vi "子VI-深度学习自动检测结果分析.vi"(2 "临界Z值":i32, 4 "临界面积百分比值":dbl, 6 "预测图片保存路径":path, 12 "产品规格":cluster{"产品长度（周长）（mm）":dbl, "产品宽度（母线长）（mm）":dbl}) -> (15 "全部检测结果":string[][](table), 16 "弥散类检测结果":string[][](table), 17 "Threshold Image":T2(plugin-control), 18 "misan":T2(plugin-control))   [LabVIEW 2018]
uses:
  <vilib>/vision/NI_Vision_Development_Module.lvlib
panel:
  out "?":string[][](table)
  in  "格式字符串 4":string="%f"
  in  "分隔符（'\\'代码显示） 3":string="\t"
  in  "Tab Control":T1
  out "?":T2(plugin-control)
  in  "格式字符串 3":string="%f"
  in  "分隔符（'\\'代码显示） 2":string="\t"
  out "弥散和分层临界灰度值":i64
  out "弥散缺陷个数":i32
  out "分层缺陷个数":i32
  out "合格？ 弥散类":string="fencengThreshold"
  out "合格？分层类":string="fencengThreshold"
  out "面积 (pixels)":i32
  in  "格式字符串 2":string="%f"
  in  "分隔符（'\\'代码显示）":string="\t"
  out "缺陷初步分类的临界值":sgl format="%#.3f"
  # "所选区域信息"
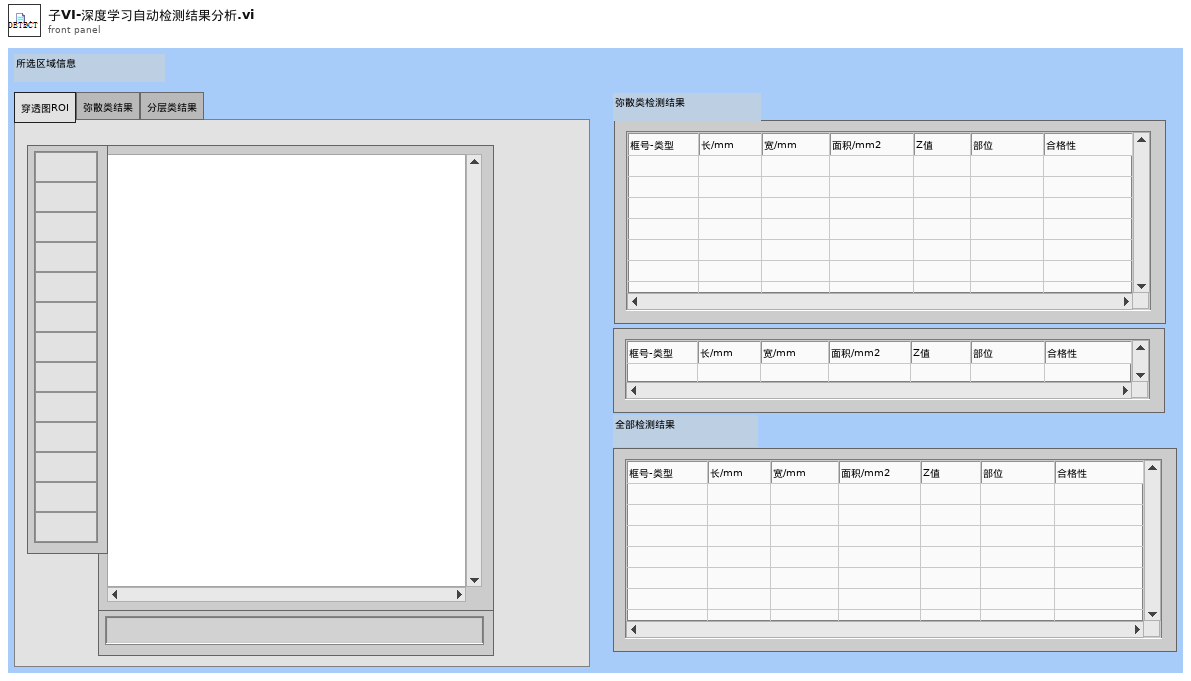
[diagram p1: front panel]
types:
  T1 = typedef "控件2.ctl" = enum32{"穿透图ROI", "弥散类结果", "分层类结果"}
  T2 = typedef "IMAQ Image.ctl" = refnum<image>
  T3 = typedef "Image Type" = u32
  T4 = typedef "Particle Parameters" = i32
  T5 = cluster{"Measurement Parameter":T4, "Range Lower Value":dbl, "Range Upper Value":dbl, "Range":bool, "Measurement Type":bool}[]
  T6 = cluster{"histogram":u32[], "Minimal Value":sgl, "Maximal Value":sgl, "Starting Value":sgl, "Interval Width":sgl, "Mean Value":sgl, "Standard  Variation":sgl, "Area (pixels)":i32}
  T7 = cluster{"Area":dbl, "Number of Holes":dbl, "Bounding Rect":cluster{"Left":dbl, "Top":dbl, "Right":dbl, "Bottom":dbl}, "Center of Mass":cluster{"X":dbl, "Y":dbl}, "Orientation":dbl, "Dimensions":cluster{"Width":dbl, "Height":dbl}}[]
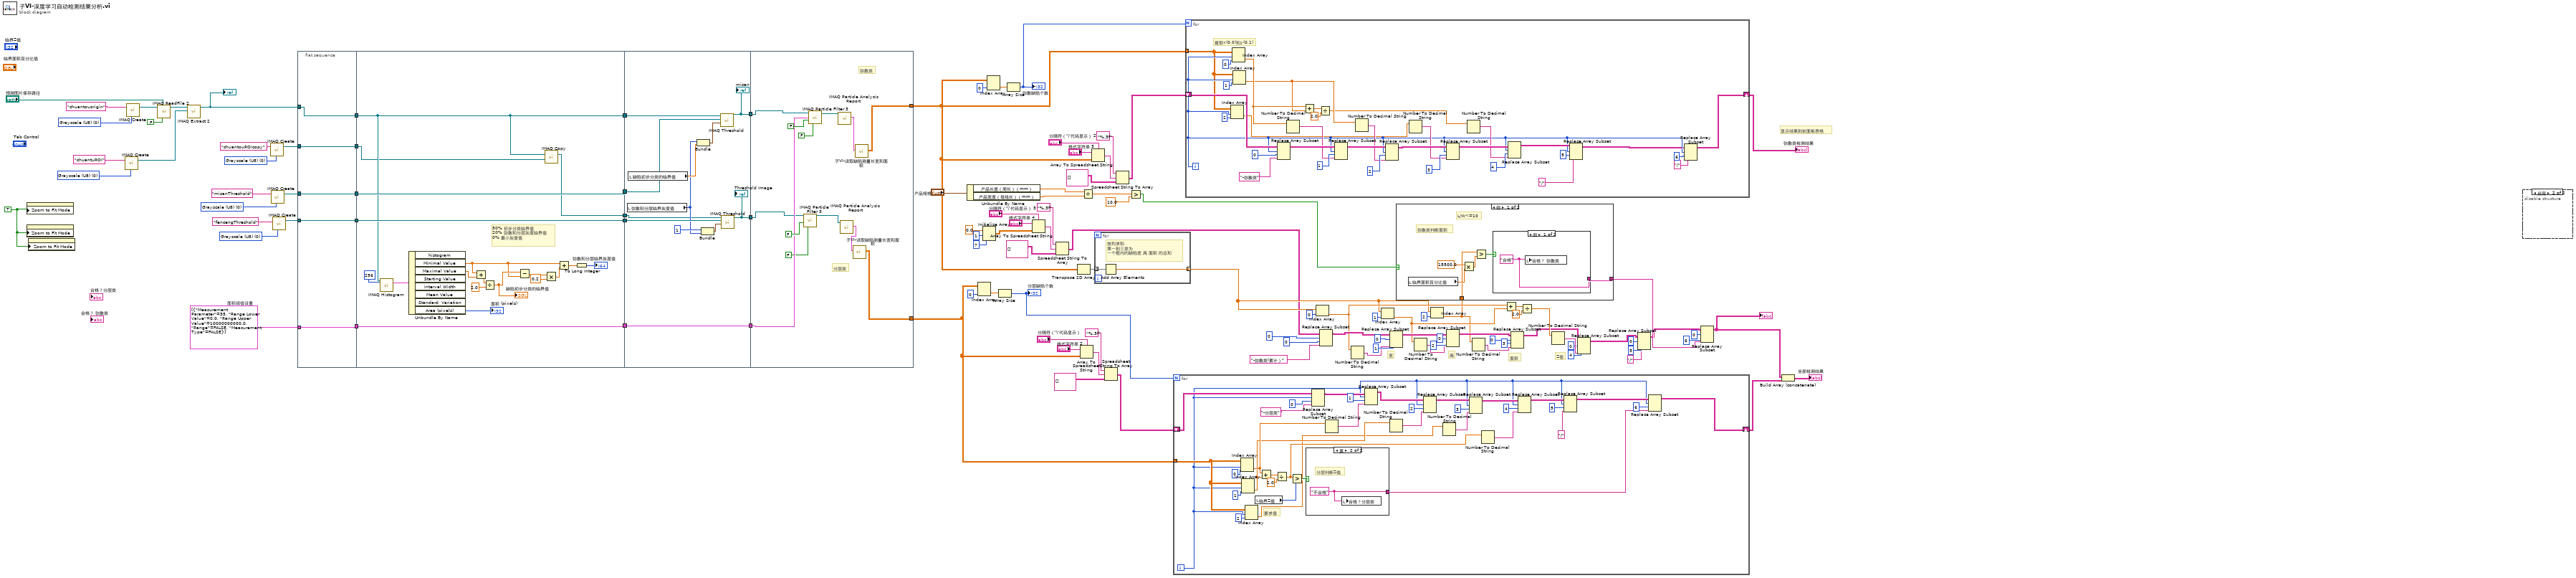
[diagram p0: block diagram]
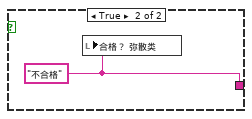
[diagram p2: hidden frame]
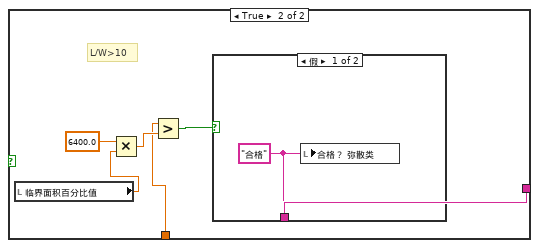
[diagram p3: hidden frame]
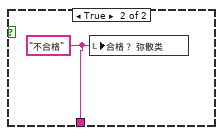
[diagram p4: hidden frame]
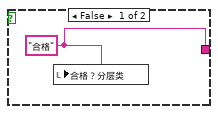
[diagram p5: hidden frame]
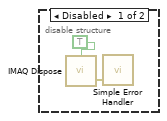
[diagram p6: hidden frame]
diagram:
  w55 = T3 0 items=["Grayscale (U8)", "Grayscale (I16)", "Grayscale (SGL)", "Complex (CSG)", "RGB (U32)", "HSL (U32)", "RGB (U64)", "Grayscale (U16)"] ("Image Type")
  w60 = TRUE ("Zoom to Fit Mode")
  w94 = T3 0 items=["Grayscale (U8)", "Grayscale (I16)", "Grayscale (SGL)", "Complex (CSG)", "RGB (U32)", "HSL (U32)", "RGB (U64)", "Grayscale (U16)"] ("Image Type")
  w95 = T3 0 items=["Grayscale (U8)", "Grayscale (I16)", "Grayscale (SGL)", "Complex (CSG)", "RGB (U32)", "HSL (U32)", "RGB (U64)", "Grayscale (U16)"] ("Image Type")
  w98 = T3 0 items=["Grayscale (U8)", "Grayscale (I16)", "Grayscale (SGL)", "Complex (CSG)", "RGB (U32)", "HSL (U32)", "RGB (U64)", "Grayscale (U16)"] ("Image Type")
  w80 = T5 [{"Measurement Parameter"=35, "Range Lower Value"=0.0, "Range Upper Value"=10000000000.0, "Range"=FALSE, "Measurement Type"=FALSE}]  # 面积阈值设置
  w111 = T3 0 items=["Grayscale (U8)", "Grayscale (I16)", "Grayscale (SGL)", "Complex (CSG)", "RGB (U32)", "HSL (U32)", "RGB (U64)", "Grayscale (U16)"] ("Image Type")
  # "显示结果到前面板表格"
  # "Z值"
  # "面积"
  # "高"
  # "宽"
  n1 = property class="ImageControl"("Zoom to Fit Mode"=w60) -> ()  [unwired: 2 in, 2 out]
  n2 = property class="ImageControl"("Zoom to Fit Mode"=w60) -> ()  [unwired: 2 in, 2 out]
  n3 = property class="ImageControl"("Zoom to Fit Mode"=w60) -> ()  [unwired: 2 in, 2 out]
  n4 = call "IMAQ Create"("Image Name"="chuantuROI", "Image Type"=w98) -> ("New Image"=w97:T2)  [unwired: 3 in, 1 out]
  n5 = call "IMAQ Create"("Image Name"="chuantouorigin", "Image Type"=w111) -> ("New Image"=w100:T2)  [unwired: 3 in, 1 out]
  n6 = call "IMAQ ReadFile 2"("Use File Path Image Type"=FALSE, "File Path"="预测图片保存路径", "Image"=w100) -> ("Image Out"=w101:T2)  [unwired: 4 in, 4 out]
  n7 = call "IMAQ Extract 2"("Image Dst"=w97, "Image Src"=w101) -> ("Image Dst Out"=w63:T2)  [unwired: 8 in, 1 out]
  "?" <- w63
  n8 = call "IMAQ Create"("Image Name"="chuantouROIcopy", "Image Type"=w55) -> ("New Image"=w58:T2)  [unwired: 3 in, 1 out]
  n9 = call "IMAQ Create"("Image Name"="misanThreshold", "Image Type"=w94) -> ("New Image"=w87:T2)  [unwired: 3 in, 1 out]
  n10 = call "IMAQ Create"("Image Name"="fencengThreshold", "Image Type"=w95) -> ("New Image"=w85:T2)  [unwired: 3 in, 1 out]
  n11 = flat-sequence {
    tunnel: w63 -> [w114]
    tunnel: w87 -> [w117]
    tunnel: [w117] -> w88
    tunnel: [w116] -> w86
    tunnel: w85 -> [w116]
    tunnel: [w115] -> w81
    tunnel: w80 -> [w115]
    tunnel: [w114] -> w61
    tunnel: w58 -> [w113]
    tunnel: [w113] -> w57
    tunnel: [w136] -> w89
    tunnel: [w135] -> w84
    tunnel: [w130] -> w79
    tunnel: w81 -> [w130]
    tunnel: w86 -> [w135]
    tunnel: w88 -> [w136]
    tunnel: [w120] -> w62
    tunnel: w61 -> [w120]
    tunnel: [w119] -> w59
    tunnel: w57 -> [w118]
    tunnel: w89 -> [w148]
    tunnel: w84 -> [w147]
    tunnel: [w138] -> w83
    tunnel: [w139] -> w82
    tunnel: w79 -> [w146]
    tunnel: [w146] -> w78
    tunnel: w62 -> [w140]
    tunnel: w59 -> [w137]
    tunnel: [w150] -> w44
    tunnel: [w152] -> w71
    tunnel: w83 -> [w156]
    tunnel: w82 -> [w155]
    tunnel: w78 -> [w159]
    frame #0 {
    }
    frame #1 {
      # "50% 初步分类临界值\n20% 弥散和分层灰度临界值\n0% 最小灰度值"
      n12 = call "IMAQ Histogram"("Number of Classes"=256, "Image"=w120) -> ("Histogram Report"=w133:T6)  [unwired: 8 in, 1 out]
      n13 = Unbundle By Name(w133) -> ("Minimal Value"=w122:sgl, "Maximal Value"=w128:sgl, "Area (pixels)"=→"面积 (pixels)":i32)  [unwired: 5 out]
      n14 = Add(x=w122, y=w128) -> (x+y=w127:sgl)
      n15 = Divide(x=w127, y=sgl 2.0) -> (x/y=w126:sgl)
      "缺陷初步分类的临界值" <- w126
      n16 = Subtract(x=w126, y=w122) -> (x-y=w124:sgl)
      n17 = Multiply(x=w124, y=0.2) -> (x*y=w123:dbl)
      n18 = call "IMAQ Copy"("Image Dst"=w118, "Image Src"=w120) -> ("Image Dst Out"=w119:T2)  [unwired: 4 in, 1 out]
      n19 = Add(x=w122, y=w123) -> (x+y=w121:dbl)
      n20 = To Long Integer(number=w121) -> (32bit integer=→"弥散和分层临界灰度值":i32)
    }
    frame #2 {
      n21 = local read "弥散和分层临界灰度值"() -> (w142:i64)
      n22 = local read "缺陷初步分类的临界值"() -> (w144:sgl)
      n23 = Bundle("弥散和分层临界灰度值"=w142, "缺陷初步分类的临界值"=w144) -> (w145:cluster{"弥散和分层临界灰度值":i64, "缺陷初步分类的临界值":sgl})  [unwired: 1 in]
      n24 = Bundle(1, "弥散和分层临界灰度值"=w142) -> (w141:cluster{i32, "弥散和分层临界灰度值":i64})  [unwired: 1 in]
      n25 = call "IMAQ Threshold"("Range"=w145, "Image Dst"=w148, "Image Src"=w140) -> ("Image Dst Out"=w139:T2)  [unwired: 3 in, 5 out]
      "misan" <- w139
      n26 = call "IMAQ Threshold"("Range"=w141, "Image Dst"=w147, "Image Src"=w137) -> ("Image Dst Out"=w138:T2)  [unwired: 3 in, 5 out]
      "Threshold Image" <- w138
    }
    frame #3 {
      # "分层类"
      # "弥散类"
      n27 = call "IMAQ Particle Filter 3"("Image Src"=w156, "Keep/Remove Particles (F)"=FALSE, "Reject Border? (F)"=FALSE) -> ("Image Dst Out"=w154:T2)  [unwired: 10 in, 2 out]
      n28 = call "IMAQ Particle Filter 3"("Image Src"=w155, "Selection Values"=w159, "Keep/Remove Particles (F)"=FALSE, "Reject Border? (F)"=FALSE) -> ("Image Dst Out"=w149:T2)  [unwired: 9 in, 2 out]
      n29 = call "IMAQ Particle Analysis Report"("Image"=w149) -> ("Particle Reports (Pixels)"=w151:T7)  [unwired: 5 in, 5 out]
      n30 = call "IMAQ Particle Analysis Report"("Image"=w154) -> ("Particle Reports (Pixels)"=w153:T7)  [unwired: 5 in, 5 out]
      n31 = call "子VI-读取缺陷测量长宽和面积.vi"("Particle Reports (Pixels)"=w153) -> ("测量结果"=w152:dbl[][])  [unwired: 10 in]
      n32 = call "子VI-读取缺陷测量长宽和面积.vi"("Particle Reports (Pixels)"=w151) -> ("测量结果"=w150:dbl[][])  [unwired: 10 in]
    }
  }
  n33 = Unbundle By Name("产品规格") -> ("产品长度（周长）（mm）"=w105:dbl, "产品宽度（母线长）（mm）"=w104:dbl)
  n34 = Index Array(array=w71, index (col)=0 ("禁用的索引 (列)")) -> (element=w93:dbl[])  [unwired: 1 in]
  n35 = Initialize Array(0.0 ("元素"), 1 ("维数大小"), 7 ("维数大小")) -> (w45:dbl[][])
  n36 = Index Array(array=w44, index (col)=0 ("禁用的索引 (列)")) -> (element=w91:dbl[])  [unwired: 1 in]
  n37 = Array Size(array=w93) -> (size(s)=w77:i32)
  "分层缺陷个数" <- w77
  n38 = Array Size(array=w91) -> (size(s)=w103:i32)
  "弥散缺陷个数" <- w103
  n39 = Array To Spreadsheet String(delimiter (Tab)="分隔符（'\\'代码显示） 3", array=w45, 3:"格式字符串 4") -> (spreadsheet string=w48:string)
  n40 = Spreadsheet String To Array(format string="%.3f", spreadsheet string=w48, array type (2D Dbl)=string[][] [] ("Array")) -> (array=w21:string[][])  [unwired: 1 in]
  n41 = Transpose 2D Array(2D array=w44) -> (transposed array=w54:dbl[][])
  n42 = Array To Spreadsheet String(delimiter (Tab)="分隔符（'\\'代码显示）", array=w71, 3:"格式字符串 2") -> (spreadsheet string=w74:string)
  n43 = Divide(x=w105, y=w104) -> (x/y=w108:dbl)
  n44 = Array To Spreadsheet String(delimiter (Tab)="分隔符（'\\'代码显示） 2", array=w44, 3:"格式字符串 3") -> (spreadsheet string=w67:string)
  n45 = for {
    tunnel: w54 -> [w163] mode=indexing
    tunnel: [w162] -> w22 mode=indexing
    # "按列求和 \n第一到三类为\n一个框内的缺陷宽 高 面积 的总和"
    n46 = Add Array Elements(numeric array=w163) -> (sum=w162:dbl)
  }
  n47 = Spreadsheet String To Array(format string="%.3f", spreadsheet string=w74, array type (2D Dbl)=string[][] [] ("Array")) -> (array=w70:string[][])  [unwired: 1 in]
  n48 = Spreadsheet String To Array(format string="%.3f", spreadsheet string=w67, array type (2D Dbl)=string[][] [] ("Array")) -> (array=w64:string[][])  [unwired: 1 in]
  n49 = Greater?(x=w108, y=10.0) -> (0:w19:bool)
  n50 = for {
    N: w77 -> [_]
    tunnel: w71 -> [w167]
    shift-right: [w176] -> w2
    shift-left: w70 -> [w185]
    i -> [w165]
    # "要求值"
    n51 = Index Array(array=w167, index (row)=w165, index (col)=0 ("禁用的索引 (列)")) -> (element=w175:dbl)
    n52 = Index Array(array=w167, index (row)=w165, index (col)=1 ("禁用的索引 (列)")) -> (element=w174:dbl)
    n53 = Index Array(array=w167, index (row)=w165, index (col)=2 ("禁用的索引 (列)")) -> (element=w164:dbl)
    n54 = local read "临界Z值"() -> (w196:i32)
    n55 = Add(x=w175, y=w174) -> (x+y=w197:dbl)
    n56 = Divide(x=w197, y=2.0) -> (x/y=w172:dbl)
    n57 = Greater?(x=w172, y=w196) -> (0:w198:bool)
    n58 = case shown="真" w198 {
      tunnel: [w199 w200] -> w171
      frame False {
        w199 = "合格" ("合格？")
        n59 = local write "合格？分层类"(w199) -> ()
      }
      frame True {
        w200 = "不合格" ("合格？")
        # "分层判断Z值"
        n60 = local write "合格？分层类"(w200) -> ()
      }
    }
    n61 = Replace Array Subset(array=w185, new element="-分层类" ("新元素/子数组"), index (row)=w165, index (col)=0 ("索引 (列)")) -> (w184:string[][])
    n62 = Number To Decimal String(number=w175) -> (decimal integer string=w183:string)  [unwired: 1 in]
    n63 = Replace Array Subset(array=w184, new element=w183, index (row)=w165, index (col)=1 ("索引 (列)")) -> (w181:string[][])
    n64 = Number To Decimal String(number=w174) -> (decimal integer string=w182:string)  [unwired: 1 in]
    n65 = Replace Array Subset(array=w181, new element=w182, index (row)=w165, index (col)=2 ("索引 (列)")) -> (w180:string[][])
    n66 = Number To Decimal String(number=w164) -> (decimal integer string=w179:string)  [unwired: 1 in]
    n67 = Replace Array Subset(array=w180, new element=w179, index (row)=w165, index (col)=3 ("索引 (列)")) -> (w178:string[][])
    n68 = Number To Decimal String(number=w172) -> (decimal integer string=w173:string)  [unwired: 1 in]
    n69 = Replace Array Subset(array=w178, new element=w173, index (row)=w165, index (col)=4 ("索引 (列)")) -> (w177:string[][])
    n70 = Replace Array Subset(array=w177, new element="/" ("新元素/子数组"), index (row)=w165, index (col)=5 ("索引 (列)")) -> (w168:string[][])
    n71 = Replace Array Subset(array=w168, new element=w171, index (row)=w165, index (col)=6 ("索引 (列)")) -> (w176:string[][])
  }
  n72 = for {
    N: w103 -> [_]
    tunnel: w44 -> [w204]
    shift-right: [w218] -> w4
    shift-left: w64 -> [w224]
    i -> [w205]
    # "提取x(0,0)和y(0,1)"
    n73 = Index Array(array=w204, index (row)=w205, index (col)=2 ("索引 (列)")) -> (element=w203:dbl)
    n74 = Index Array(array=w204, index (row)=w205, index (col)=0 ("禁用的索引 (列)")) -> (element=w212:dbl)
    n75 = Index Array(array=w204, index (row)=w205, index (col)=1 ("禁用的索引 (列)")) -> (element=w211:dbl)
    n76 = Replace Array Subset(array=w224, new element="-弥散类" ("新元素/子数组"), index (row)=w205, index (col)=0 ("索引 (列)")) -> (w223:string[][])
    n77 = Number To Decimal String(number=w212) -> (decimal integer string=w217:string)  [unwired: 1 in]
    n78 = Add(x=w212, y=w211) -> (x+y=w214:dbl)
    n79 = Divide(x=w214, y=2.0) -> (x/y=w210:dbl)
    n80 = Replace Array Subset(array=w223, new element=w217, index (row)=w205, index (col)=1 ("索引 (列)")) -> (w222:string[][])
    n81 = Number To Decimal String(number=w211) -> (decimal integer string=w216:string)  [unwired: 1 in]
    n82 = Replace Array Subset(array=w222, new element=w216, index (row)=w205, index (col)=2 ("索引 (列)")) -> (w221:string[][])
    n83 = Number To Decimal String(number=w203) -> (decimal integer string=w215:string)  [unwired: 1 in]
    n84 = Replace Array Subset(array=w221, new element=w215, index (row)=w205, index (col)=3 ("索引 (列)")) -> (w220:string[][])
    n85 = Number To Decimal String(number=w210) -> (decimal integer string=w209:string)  [unwired: 1 in]
    n86 = Replace Array Subset(array=w220, new element=w209, index (row)=w205, index (col)=4 ("索引 (列)")) -> (w219:string[][])
    n87 = Replace Array Subset(array=w219, new element="/" ("新元素/子数组"), index (row)=w205, index (col)=5 ("索引 (列)")) -> (w202:string[][])
    n88 = Replace Array Subset(array=w202, new element="/" ("新元素/子数组"), index (row)=w205, index (col)=6 ("索引 (列)")) -> (w218:string[][])
  }
  "弥散类检测结果" <- w4
  n89 = Index Array(array=w22, index=0 ("索引")) -> (element=w24:dbl)
  n90 = Replace Array Subset(array=w21, new element="-弥散类(累计）" ("新元素/子数组"), index (row)=0 ("禁用的索引 (行)"), index (col)=0 ("索引 (列)")) -> (w38:string[][])
  n91 = Number To Decimal String(number=w24) -> (decimal integer string=w37:string)  [unwired: 1 in]
  n92 = Index Array(array=w22, index=1 ("索引")) -> (element=w23:dbl)
  n93 = Replace Array Subset(array=w38, new element=w37, index (row)=0 ("索引 (行)"), index (col)=1 ("索引 (列)")) -> (w35:string[][])
  n94 = Number To Decimal String(number=w23) -> (decimal integer string=w28:string)  [unwired: 1 in]
  n95 = Index Array(array=w22, index=2 ("索引")) -> (element=w18:dbl)
  n96 = case shown="假" w19 {
    tunnel: [w238 w246] -> w6
    tunnel: w18 -> [w234 w242]
    frame False {
      # "弥散类判断面积"
      # "L/W<=10"
      n97 = local read "临界面积百分比值"() -> (w236:dbl)
      n98 = Multiply(x=15500.0, y=w236) -> (x*y=w235:dbl)
      n99 = Greater?(x=w234, y=w235) -> (0:w239:bool)
      n100 = case shown="假" w239 {
        tunnel: [w240 w241] -> w238
        frame False {
          w240 = "合格" ("合格？")
          n101 = local write "合格？ 弥散类"(w240) -> ()
        }
        frame True {
          w241 = "不合格" ("合格？")
          n102 = local write "合格？ 弥散类"(w241) -> ()
        }
      }
    }
    frame True {
      # "L/W>10"
      n103 = local read "临界面积百分比值"() -> (w243:dbl)
      n104 = Multiply(x=6400.0, y=w243) -> (x*y=w245:dbl)
      n105 = Greater?(x=w242, y=w245) -> (0:w247:bool)
      n106 = case shown="假" w247 {
        tunnel: [w248 w249] -> w246
        frame False {
          w248 = "合格" ("合格？")
          n107 = local write "合格？ 弥散类"(w248) -> ()
        }
        frame True {
          w249 = "不合格" ("合格？")
          n108 = local write "合格？ 弥散类"(w249) -> ()
        }
      }
    }
  }
  n109 = Replace Array Subset(array=w35, new element=w28, index (row)=0 ("索引 (行)"), index (col)=2 ("禁用的索引 (列)")) -> (w30:string[][])
  n110 = Number To Decimal String(number=w18) -> (decimal integer string=w27:string)  [unwired: 1 in]
  n111 = Add(x=w24, y=w23) -> (x+y=w26:dbl)
  n112 = Replace Array Subset(array=w30, new element=w27, index (row)=0 ("索引 (行)"), index (col)=3 ("索引 (列)")) -> (w13:string[][])
  n113 = Divide(x=w26, y=2.0) -> (x/y=w14:dbl)
  n114 = Number To Decimal String(number=w14) -> (decimal integer string=w17:string)  [unwired: 1 in]
  n115 = Replace Array Subset(array=w13, new element=w17, index (row)=0 ("索引 (行)"), index (col)=4 ("索引 (列)")) -> (w10:string[][])
  n116 = Replace Array Subset(array=w10, new element="/" ("新元素/子数组"), index (row)=0 ("索引 (行)"), index (col)=5 ("索引 (列)")) -> (w5:string[][])
  n117 = Replace Array Subset(array=w5, new element=w6, index (row)=0 ("索引 (行)"), index (col)=6 ("索引 (列)")) -> (w1:string[][])
  "?" <- w1
  n118 = Build Array (concatenate)(w1, w2) -> (→"全部检测结果":string[][])
  n119 = disable-structure shown="启用" {
    frame Disabled {
      n120 = call "IMAQ Dispose"("All Images? (No)"=TRUE) -> ("error out"=w251:errorcluster)  [unwired: 5 in]
      n121 = call <vilib>:"Simple Error Handler.vi"("error in (no error)"=w251) -> ()  [unwired: 4 in, 5 out]
    }
    frame Enabled {
    }
  }
